vi "Migrate Measurement Dependencies.vi"(0 "Project path":path, 1 "Init":T1[](array[typedef]), 5 "Measurement path":path, 7 "Dependencies path":path[](array[path]), 9 "Plug-in name":string, 11 "error in (no error)":errorcluster) -> (4 "Project reference":refnum<vi>, 6 "MeasurementCore reference":refnum<vi>, 8 "Outside items":string[](array[string]), 15 "error out":errorcluster)   [LabVIEW 2021, in "Multiple Converter.lvlib"]
uses:
  Multiple Converter.lvlib
  controls/Library Info.ctl
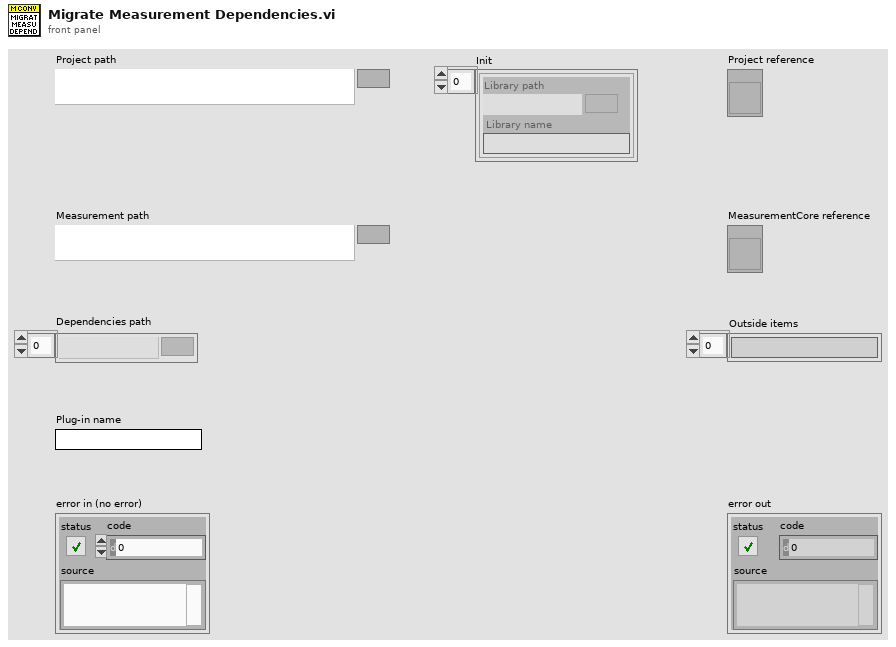
[diagram p1: front panel]
types:
  T1 = typedef "Multiple Converter.lvlib/Library Info.ctl" = cluster{"Library path":path, "Library name":string}
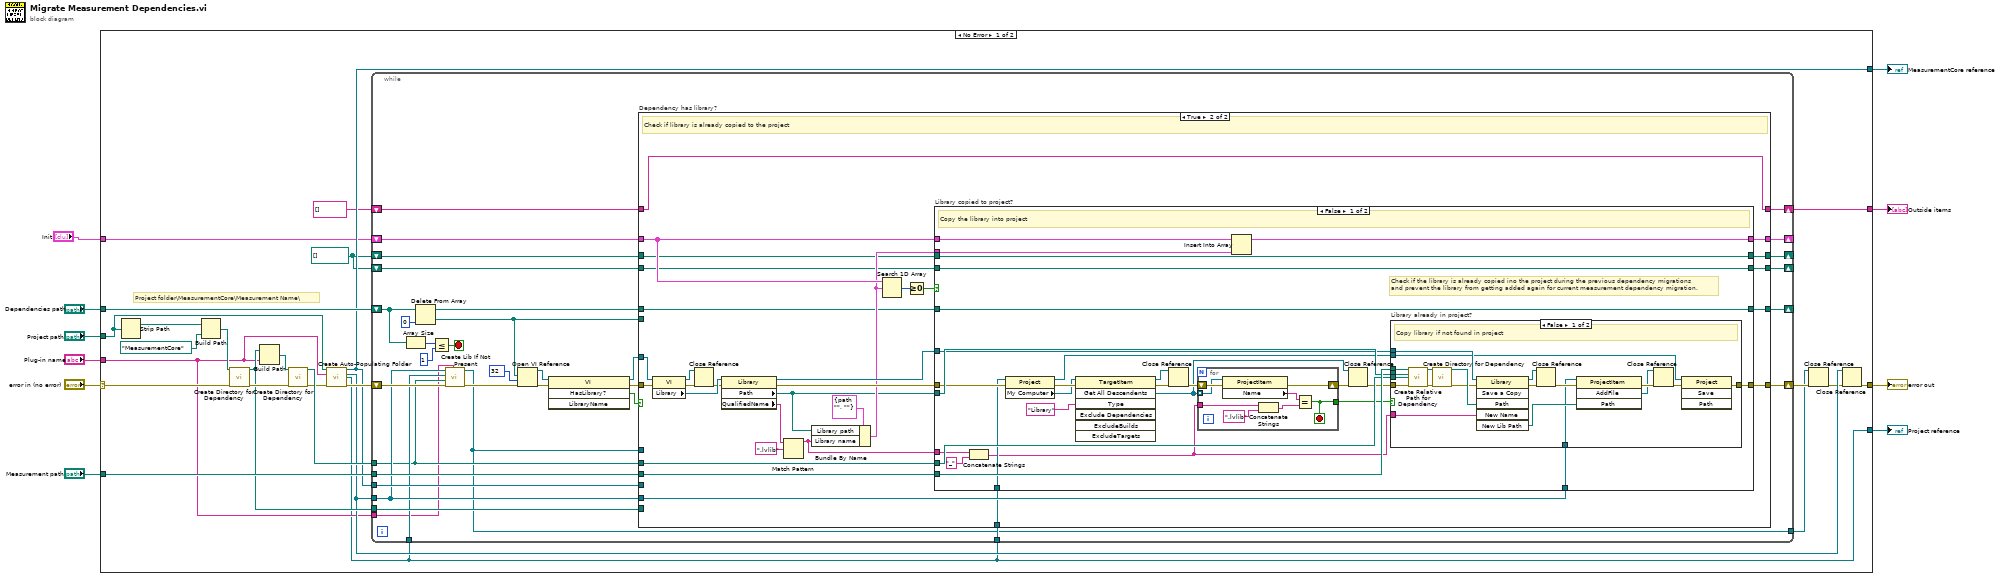
[diagram p0: block diagram]
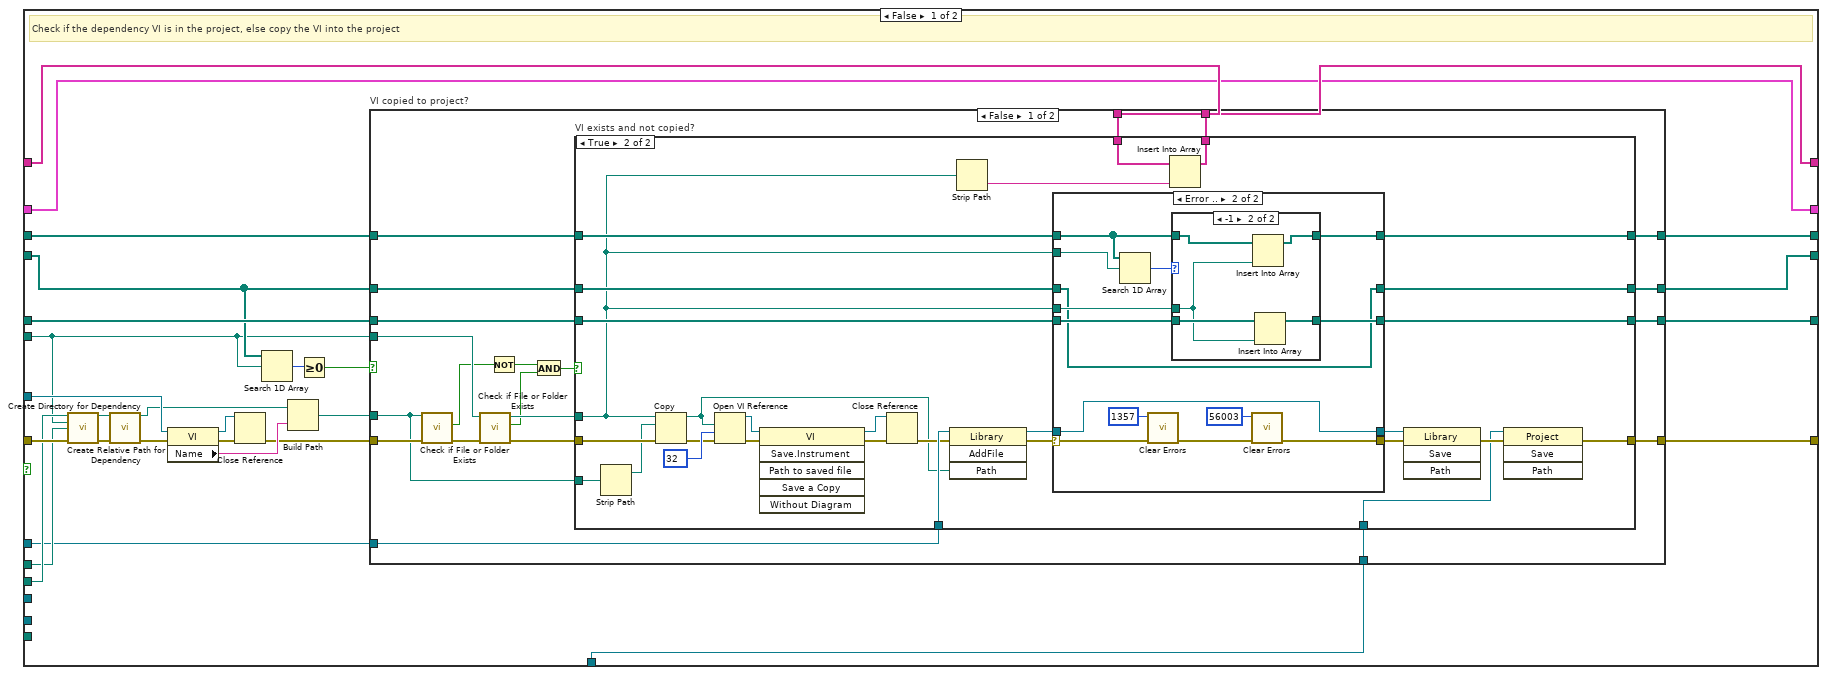
[diagram p2: hidden frame]
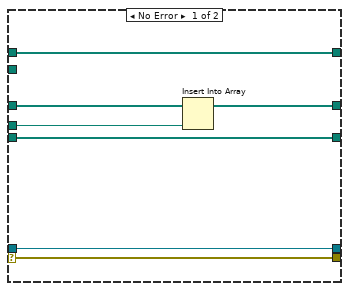
[diagram p4: hidden frame]
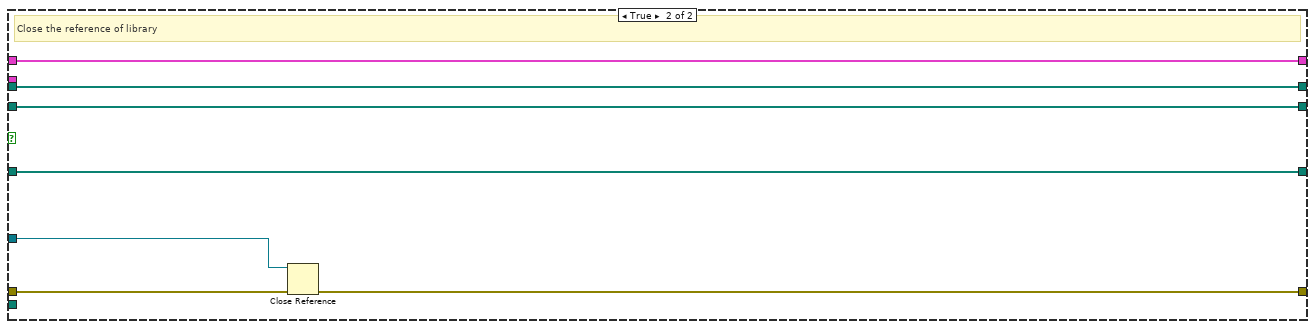
[diagram p8: hidden frame]
diagram:
  n1 = case shown="No Error" "error in (no error)" {
    selector: "error in (no error)" -> [w27 w280]
    tunnel: [w20 w280] -> w9
    tunnel: "Project path" -> [w26 _]
    tunnel: "Measurement path" -> [w31 _]
    tunnel: "Dependencies path" -> [w35 _]
    tunnel: "Plug-in name" -> [w18 _]
    tunnel: [w22 _] -> w4
    tunnel: [w15 _] -> w3
    tunnel: [w16 _] -> w2
    tunnel: "Init" -> [w11 _]
    frame No Error {
      w12 = path[] []
      # "Project folder\\MeasurementCore\\Measurement Name\\"
      n2 = Strip Path(path=w26) -> (stripped path=w30:path)  [unwired: 1 out]
      n3 = Build Path(base path=w30, name or relative path=path "MeasurementCore") -> (appended path=w28:path)
      n4 = call "Create Directory for Dependency.vi"("Directory path"=w28, "error in (no error)"=w27) -> ("Directory path out"=w21:path, "error out"=w25:errorcluster)  [unwired: 12 in]
      n5 = Build Path(base path=w21, name or relative path=w18) -> (appended path=w34:path)
      n6 = call "Create Directory for Dependency.vi"("Directory path"=w34, "error in (no error)"=w25) -> ("Directory path out"=w33:path, "error out"=w24:errorcluster)  [unwired: 12 in]
      n7 = call "Create Auto-Populating Folder.vi"("Project path"=w26, "Plug-in name"=w18, "error in (no error)"=w24) -> ("MeasurementCore reference"=w22:refnum<vi>, "Folder reference"=w19:refnum<vi>, "Project reference"=w15:refnum<vi>, "error out"=w23:errorcluster)  [unwired: 9 in]
      n8 = while {
        shift-right: [w57] -> w32
        shift-left: w23 -> [w45]
        shift-right: [w50] -> _
        shift-left: w35 -> [w67]
        tunnel: w33 -> [w41]
        shift-right: [w56] -> _
        shift-left: w11 -> [w59]
        tunnel: w31 -> [w55]
        shift-right: [w52] -> _
        shift-left: w12 -> [w53]
        tunnel: w22 -> [w49]
        tunnel: w21 -> [w48]
        tunnel: w19 -> [w43]
        tunnel: w18 -> [w40]
        shift-right: [w46] -> w16
        shift-left: string[] [] -> [w47]
        tunnel: w15 -> [w42]
        tunnel: w15 -> [w39]
        shift-right: [w38] -> _
        shift-left: w12 -> [w37]
        tunnel: [w36] -> w13
        stop <- w66 stop-if-true
        n9 = Array Size(array=w67) -> (size(s)=w69:i32)
        n10 = Delete From Array(array=w67, index=0) -> (deleted portion=w54:path, array with subset deleted=w51:path[])  [unwired: 1 in]
        n11 = Less Or Equal?(x=w69, y=1) -> (x <= y?=w66:bool)
        n12 = call "Create Lib If Not Present.vi"("Plug-in name"=w40, "error in (no error)"=w45, "DestDirectory"=w41, "ProjectRef"=w42, "VirtualFolderRef"=w43) -> ("error out"=w44:errorcluster, "Library Refnum"=w36:refnum<vi>)  [unwired: 5 in]
        n13 = Open VI Reference(vi path=w54, options=32, error in (no error)=w44) -> (vi reference=w63:refnum<vi>, error out=w65:errorcluster)  [unwired: 3 in]
        n14 = invoke class="VI" method="HasLibrary?"(reference=w63, error in=w65) -> (reference out=w60:refnum<vi>, error out=w61:errorcluster, "Has Library?"=w62:bool)  [unwired: 2 in, 1 out]
        n15 = case "Dependency has library?" shown="True" w62 {
          tunnel: w61 -> [w96 w214]
          tunnel: w60 -> [w92 w215]
          tunnel: w59 -> [w73 w202]
          tunnel: [w87 w203] -> w57
          tunnel: [w73 w201] -> w56
          tunnel: w55 -> [w95 w199]
          tunnel: w41 -> [w78 w197]
          tunnel: w54 -> [w82 _]
          tunnel: w53 -> [w83 w194]
          tunnel: [w77 w193] -> w52
          tunnel: w51 -> [w86 w192]
          tunnel: [w85 w191] -> w50
          tunnel: w49 -> [_ _]
          tunnel: w48 -> [_ _]
          tunnel: w43 -> [_ w190]
          tunnel: w47 -> [w75 w189]
          tunnel: [w74 w189] -> w46
          tunnel: w36 -> [w76 _]
          tunnel: w39 -> [w70 w188]
          tunnel: [w72 w186] -> w38
          tunnel: w37 -> [w71 w187]
          frame False {
            # "Check if the dependency VI is in the project, else copy the VI into the project"
            n16 = call "Create Relative Path for Dependency.vi"("Old Main Path"=w95, "Old Dependency Path"=w82, "New Dir"=w78, "error in (no error)"=w96) -> ("Directory"=w94:path, "error out"=w97:errorcluster)  [unwired: 10 in]
            n17 = call "Create Directory for Dependency.vi"("Directory path"=w94, "error in (no error)"=w97) -> ("Directory path out"=w84:path, "error out"=w93:errorcluster)  [unwired: 12 in]
            n18 = property class="VI"(reference=w92, error in=w93) -> (reference out=w88:refnum<vi>, error out=w91:errorcluster, "Name"=w90:string)
            n19 = Close Reference(reference=w88, error in (no error)=w91) -> (error out=w89:errorcluster)
            n20 = Search 1D Array(1D array=w83, element=w82) -> (index of element=w81:i32)  [unwired: 1 in]
            n21 = Build Path(base path=w84, name or relative path=w90) -> (appended path=w80:path)
            n22 = Greater Or Equal To 0?(x=w81) -> (x >= 0?=w79:bool)
            n23 = case "VI copied to project?" shown="False" w79 {
              tunnel: w89 -> [w118 w185]
              tunnel: w82 -> [w117 _]
              tunnel: [w114 w185] -> w87
              tunnel: w83 -> [w113 w184]
              tunnel: [w112 w184] -> w77
              tunnel: w80 -> [w108 _]
              tunnel: w86 -> [w111 w183]
              tunnel: [w110 w183] -> w85
              tunnel: w75 -> [w103 w182]
              tunnel: [w102 w182] -> w74
              tunnel: w76 -> [w101 _]
              tunnel: [w100 w181] -> w72
              tunnel: w71 -> [w99 w181]
              tunnel: w70 -> [w98 _]
              frame False {
                n24 = call <vilib>:"Check if File or Folder Exists.vi"("error in (no error)"=w118, "path"=w108) -> ("error out"=w109:errorcluster, "file or folder exists?"=w107:bool)  [unwired: 7 in, 1 out]
                n25 = call <vilib>:"Check if File or Folder Exists.vi"("error in (no error)"=w109, "path"=w117) -> ("error out"=w116:errorcluster, "file or folder exists?"=w105:bool, "dup path"=w115:path)  [unwired: 7 in]
                n26 = Not(x=w107) -> (.not. x?=w106:bool)
                n27 = And(x=w106, y=w105) -> (x .and. y?=w104:bool)
                n28 = case "VI exists and not copied?" shown="True" w104 {
                  tunnel: w116 -> [w123 w152]
                  tunnel: w115 -> [_ w132]
                  tunnel: [w123 w134] -> w114
                  tunnel: w113 -> [w122 w151]
                  tunnel: [w122 w150] -> w112
                  tunnel: w108 -> [_ w147]
                  tunnel: w111 -> [w121 w136]
                  tunnel: [w121 w135] -> w110
                  tunnel: w103 -> [w120 w146]
                  tunnel: [w120 w144] -> w102
                  tunnel: w101 -> [_ w143]
                  tunnel: [w119 w142] -> w100
                  tunnel: w99 -> [w119 w141]
                  tunnel: w98 -> [_ w133]
                  frame False {
                  }
                  frame True {
                    n29 = Strip Path(path=w147) -> (stripped path=w149:path)  [unwired: 1 out]
                    n30 = Copy(8:w152, 10:w149, 11:w132) -> (0:w126:errorcluster, 3:w124:path)  [unwired: 2 in, 1 out]
                    n31 = Open VI Reference(vi path=w124, options=32, error in (no error)=w126) -> (vi reference=w129:refnum<vi>, error out=w130:errorcluster)  [unwired: 3 in]
                    n32 = invoke class="VI" method="Save.Instrument"(reference=w129, error in=w130) -> (reference out=w127:refnum<vi>, error out=w128:errorcluster)  [unwired: 4 in, 4 out]
                    n33 = Close Reference(reference=w127, error in (no error)=w128) -> (error out=w125:errorcluster)
                    n34 = invoke class="Library" method="AddFile"(reference=w143, error in=w125, "Path"=w124) -> (reference out=w140:refnum<vi>, error out=w139:errorcluster)  [unwired: 1 in, 2 out]
                    n35 = Strip Path(path=w132) -> (name=w145:string)  [unwired: 1 out]
                    n36 = case shown="Error .." w139 {
                      selector: w139 -> [w154 w173]
                      tunnel: w151 -> [w159 w160]
                      tunnel: [w158 w160] -> w150
                      tunnel: w132 -> [w157 w163]
                      tunnel: [w156 w164] -> w142
                      tunnel: w141 -> [w156 w165]
                      tunnel: [w155 w162] -> w137
                      tunnel: w140 -> [w155 w162]
                      tunnel: [w154 w171] -> w138
                      tunnel: w136 -> [w153 w167]
                      tunnel: [w153 w166] -> w135
                      tunnel: w132 -> [_ w168]
                      frame No Error {
                        n37 = Insert Into Array(array=w159, new element=w157) -> (w158:path[])  [unwired: 1 in]
                      }
                      frame Error {
                        n38 = Search 1D Array(1D array=w165, element=w168) -> (index of element=w161:i32)  [unwired: 1 in]
                        n39 = call <vilib>:"Clear Errors.vi"("error in (no error)"=w173, "specific error code to clear (0: all)"=1357) -> ("error out"=w172:errorcluster)  [unwired: 4 in, 1 out]
                        n40 = case shown="-1" w161 {
                          tunnel: w167 -> [w174 w180]
                          tunnel: [w174 w179] -> w166
                          tunnel: w165 -> [w175 w178]
                          tunnel: [w175 w177] -> w164
                          tunnel: w163 -> [_ w176]
                          frame Default {
                          }
                          frame -1 {
                            n41 = Insert Into Array(array=w178, new element=w176) -> (w177:path[])  [unwired: 1 in]
                            n42 = Insert Into Array(array=w180, new element=w176) -> (w179:path[])  [unwired: 1 in]
                          }
                        }
                        n43 = call <vilib>:"Clear Errors.vi"("error in (no error)"=w172, "specific error code to clear (0: all)"=56003) -> ("error out"=w171:errorcluster)  [unwired: 4 in, 1 out]
                      }
                    }
                    n44 = Insert Into Array(array=w146, new element=w145) -> (w144:string[])  [unwired: 1 in]
                    n45 = invoke class="Library" method="Save"(reference=w137, error in=w138) -> (error out=w148:errorcluster)  [unwired: 2 in, 3 out]
                    n46 = invoke class="Project" method="Save"(reference=w133, error in=w148) -> (error out=w134:errorcluster)  [unwired: 2 in, 3 out]
                  }
                }
              }
              frame True {
              }
            }
          }
          frame True {
            # "Check if library is already copied to the project"
            n47 = property class="VI"(reference=w215, error in=w214) -> (reference out=w205:refnum<vi>, error out=w213:errorcluster, "Library"=w212:refnum<vi>)
            n48 = Close Reference(reference=w205, error in (no error)=w213) -> (error out=w206:errorcluster)
            n49 = property class="Library"(reference=w212, error in=w206) -> (reference out=w204:refnum<vi>, error out=w207:errorcluster, "Path"=w198:path, "QualifiedName"=w208:string)
            n50 = Match Pattern(string=w208, regular expression=".lvlib") -> (before substring=w195:string)  [unwired: 1 in, 3 out]
            n51 = Bundle By Name(cluster=T1 {"Library path"=path "", "Library name"=""} ("Cluster"), "Library path"=w198, "Library name"=w195) -> (w200:T1)
            n52 = Search 1D Array(1D array=w202, element=w200) -> (index of element=w210:i32)  [unwired: 1 in]
            n53 = Greater Or Equal To 0?(x=w210) -> (x >= 0?=w209:bool)
            n54 = case "Library copied to project?" shown="False" w209 {
              tunnel: w207 -> [w229 w278]
              tunnel: w204 -> [w237 w279]
              tunnel: [w231 w277] -> w203
              tunnel: w202 -> [w243 w276]
              tunnel: [w242 w276] -> w201
              tunnel: w200 -> [w241 _]
              tunnel: w199 -> [w240 _]
              tunnel: w198 -> [w239 _]
              tunnel: w197 -> [w238 _]
              tunnel: w195 -> [w233 _]
              tunnel: w194 -> [w236 w275]
              tunnel: [w236 w275] -> w193
              tunnel: [w235 w274] -> w191
              tunnel: w192 -> [w235 w274]
              tunnel: w190 -> [w234 _]
              tunnel: w188 -> [w228 _]
              tunnel: [w230 w273] -> w186
              tunnel: w187 -> [w230 w273]
              frame False {
                # "Check if the library is already copied ino the project during the previous dependency migrations \nand prevent the library from getting added again for current measurement dependency migration."
                # "Copy the library into project"
                n55 = Concatenate Strings(w233, "_" ("string")) -> (w223:string)
                n56 = property class="Project"(reference=w228, error in=w229) -> (reference out=w225:refnum<vi>, error out=w227:errorcluster, "My Computer"=w226:refnum<vi>)
                n57 = invoke class="TargetItem" method="Get All Descendents"(reference=w226, error in=w227, "Type"="Library") -> (reference out=w220:refnum<vi>, error out=w222:errorcluster, "All Descendents"=w217:refnum<vi>[])  [unwired: 4 in, 4 out]
                n58 = Close Reference(reference=w220, error in (no error)=w222) -> (error out=w221:errorcluster)
                n59 = for {
                  shift-right: [w271] -> w219
                  shift-left: w221 -> [w272]
                  tunnel: w217 -> [w270] mode=indexing
                  tunnel: w223 -> [w265]
                  tunnel: [w268] -> w216
                  stop <- w268 stop-if-true
                  n60 = property class="ProjectItem"(reference=w270, error in=w272) -> (error out=w271:errorcluster, "Name"=w269:string)  [unwired: 1 out]
                  n61 = Concatenate Strings(w265, ".lvlib" ("string")) -> (w266:string)
                  n62 = Equal?(x=w269, y=w266) -> (x = y?=w268:bool)
                }
                n63 = Insert Into Array(array=w243, new element=w241) -> (w242:T1[])  [unwired: 1 in]
                n64 = Close Reference(reference=w217, error in (no error)=w219) -> (error out=w218:errorcluster)
                n65 = case "Library already in project?" shown="False" w216 {
                  tunnel: w240 -> [w261 _]
                  tunnel: w239 -> [w260 _]
                  tunnel: w238 -> [w259 _]
                  tunnel: w237 -> [w255 _]
                  tunnel: w234 -> [w248 _]
                  tunnel: [w247 w264] -> w231
                  tunnel: w225 -> [w246 _]
                  tunnel: w223 -> [w245 _]
                  tunnel: w218 -> [w244 w264]
                  frame False {
                    # "Copy library if not found in project"
                    n66 = call "Create Relative Path for Dependency.vi"("Old Main Path"=w261, "Old Dependency Path"=w260, "New Dir"=w259, "error in (no error)"=w244) -> ("Directory"=w257:path, "error out"=w258:errorcluster)  [unwired: 10 in]
                    n67 = call "Create Directory for Dependency.vi"("Directory path"=w257, "error in (no error)"=w258) -> ("Directory path out"=w256:path, "error out"=w254:errorcluster)  [unwired: 12 in]
                    n68 = invoke class="Library" method="Save a Copy"(reference=w255, error in=w254, "Path"=w256, "New Name"=w245) -> (reference out=w262:refnum<vi>, error out=w263:errorcluster, "New Lib Path"=w251:path)  [unwired: 2 in, 3 out]
                    n69 = Close Reference(reference=w262, error in (no error)=w263) -> (error out=w253:errorcluster)
                    n70 = invoke class="ProjectItem" method="AddFile"(reference=w248, error in=w253, "Path"=w251) -> (error out=w252:errorcluster, "AddFile"=w249:refnum<vi>)  [unwired: 1 in, 2 out]
                    n71 = Close Reference(reference=w249, error in (no error)=w252) -> (error out=w250:errorcluster)
                    n72 = invoke class="Project" method="Save"(reference=w246, error in=w250) -> (error out=w247:errorcluster)  [unwired: 2 in, 3 out]
                  }
                  frame True {
                  }
                }
              }
              frame True {
                # "Close the reference of library"
                n73 = Close Reference(reference=w279, error in (no error)=w278) -> (error out=w277:errorcluster)
              }
            }
          }
        }
      }
      n74 = Close Reference(reference=w13, error in (no error)=w32) -> (error out=w14:errorcluster)
      n75 = Close Reference(reference=w19, error in (no error)=w14) -> (error out=w20:errorcluster)
    }
    frame Error {
    }
  }
  "error out" <- w9
  "MeasurementCore reference" <- w4
  "Project reference" <- w3
  "Outside items" <- w2
